vi "Sensorer_Cop.vi"() -> ()   [LabVIEW 2019]
uses:
  <vilib>/myRIO/Instrument Drivers/Onboard IO/AI/typedefs/AI Reference.ctl
  <vilib>/myRIO/Common/Instrument Driver Framework/Utilities/typedefs/myRIO Generic Hardware Reference.ctl
  <vilib>/myRIO/Common/Instrument Driver Framework/Utilities/typedefs/Hardware Version Enum.ctl
  <vilib>/myRIO/Common/Instrument Driver Framework/Utilities/typedefs/myRIO v1.0 Reference.ctl
  <vilib>/myRIO/Common/Instrument Driver Framework/Utilities/typedefs/Generic FPGA Reference.ctl
  <vilib>/myRIO/Common/Instrument Driver Framework/myRIO v1.0/AI/typedefs/AI Channels List.ctl
  <vilib>/myRIO/Common/Instrument Driver Framework/myRIO v1.0/AI/typedefs/AI Channels Enum.ctl
  <vilib>/myRIO/Common/Instrument Driver Framework/Utilities/typedefs/Analog Scaling Constants List.ctl
  <vilib>/myRIO/Common/Instrument Driver Framework/Utilities/typedefs/Analog Scaling Constants.ctl
  <vilib>/userDefined/High Color/nirio_resource_hc.ctl
  <vilib>/myRIO/Common/Instrument Driver Framework/Utilities/vis/Is FPGA Ref Available.vi
  <vilib>/myRIO/Common/Instrument Driver Framework/myRIO v1.0/AI/vis/myRIO v1.1 Open AI.vi
  <vilib>/myRIO/Instrument Drivers/Onboard IO/AI/vis/Read.vi
  <vilib>/myRIO/Common/Instrument Driver Framework/Utilities/vis/Validate Channels.vi
  <vilib>/myRIO/Common/Instrument Driver Framework/myRIO v1.0/AI/vis/myRIO v1.0 Reserve AI.vi
  <vilib>/myRIO/Common/Instrument Driver Framework/myRIO v1.0/AI/vis/myRIO v1.0 Build MUX Configuration AI.vi
  <vilib>/myRIO/Common/Instrument Driver Framework/myRIO v1.0/Resource Manager/vis/myRIO v1.0 Reserve Channel List.vi
  <vilib>/myRIO/Common/Instrument Driver Framework/myRIO v1.0/Resource Manager/vis/myRIO v1.0 Reserve Channel.vi
  <vilib>/myRIO/Common/Instrument Driver Framework/myRIO v1.0/Resource Manager/vis/myRIO v1.0 Unreserve Channel.vi
  <vilib>/myRIO/Common/Instrument Driver Framework/myRIO v1.0/Resource Manager/vis/myRIO v1.0 Build Mutex Name.vi
  <vilib>/Utility/VariantDataType/GetNumericInfo.vi
  <vilib>/Utility/error.llb/Error Cluster From Error Code.vi
  <vilib>/myRIO/Common/Instrument Driver Framework/myRIO v1.0/myRIO v1.1 Open.vi
  <vilib>/myRIO/Common/Instrument Driver Framework/myRIO v1.0/AI/vis/myRIO v1.0 Get Scaling Constants AI.vi
  <vilib>/myRIO/Common/Instrument Driver Framework/Utilities/vis/IO Manager.vi
  <vilib>/myRIO/Common/Instrument Driver Framework/Utilities/vis/Configuration Manager.vi
  <vilib>/myRIO/Common/Instrument Driver Framework/myRIO v1.0/myRIO v1.0 Close.vi
  <vilib>/myRIO/Common/Instrument Driver Framework/myRIO v1.0/AI/vis/myRIO v1.0 Read AI.vi
  <vilib>/myRIO/Express VI/Onboard IO/AI/AI Express VI.xnode
  <vilib>/myRIO/Instrument Drivers/Onboard IO/AI/vis/myRIO AI Open.xnode
  <vilib>/myRIO/Instrument Drivers/Onboard IO/AI/AI.lvlib
panel:
  in  "x Left":dbl[](array[numeric])
  in  "kal left":dbl
  in  "kal Right":dbl
  in  "x Right":dbl[](array[numeric])
  out "Cop Right":cluster{dbl[], dbl[]}(graph)
  out "Cop Left":cluster{dbl[], dbl[]}(graph)
  out "x(F.L)":dbl
  out "y(F.L)":dbl
  out "Sum (F.L)":dbl
  out "sum(F.R)":dbl
  out "y(F.R)":dbl
  out "x(F.R)":dbl
  in  "Cal(F.R)":dbl[](array[numeric])
  out "Kg (R)":dbl[](array[numeric])
  out "Sum(R)":dbl
  out "Sum(L)":dbl
  out "Kg(L)":dbl[](array[numeric])
  in  "Cal(F.L)":dbl[](array[numeric])
  out "Sensor 10":dbl=0.0038137989155123176 format="%0.5f"
  out "Axial(R)":T1(graph)
  out "Sensor 9":dbl=0.0038137989155123176 format="%0.5f"
  out "Axial(L)":T1(graph)
  out "Sensor 8":dbl=0.0038137989155123176 format="%0.5f"
  out "Back Right(F.R)":T1(graph)
  out "Sensor 7":dbl=0.0038137989155123176 format="%0.5f"
  out "Back Left(F.R)":T1(graph)
  out "Front Right(F.R)":T1(graph)
  out "Sensor 6":dbl=0.0038137989155123176 format="%0.5f"
  out "Front Left(F.R)":T1(graph)
  out "Sensor 5":dbl=0.0038137989155123176 format="%0.5f"
  out "Back Right(F.L)":T1(graph)
  out "Sensor 4":dbl=0.0038137989155123176 format="%0.5f"
  out "Back Left(F.L)":T1(graph)
  out "Sensor 3":dbl=0.0038137989155123176 format="%0.5f"
  out "Front  Right(F.L)":T1(graph)
  out "Sensor 2":dbl=0.0038137989155123176 format="%0.5f"
  in  "STOP SYSTEM":bool
  in  "ZERO ALL SENSORS":bool
  out "Sensor 1":dbl=0.0038137989155123176 format="%0.5f"
  out "Front  Left(F.L)":T1(graph)
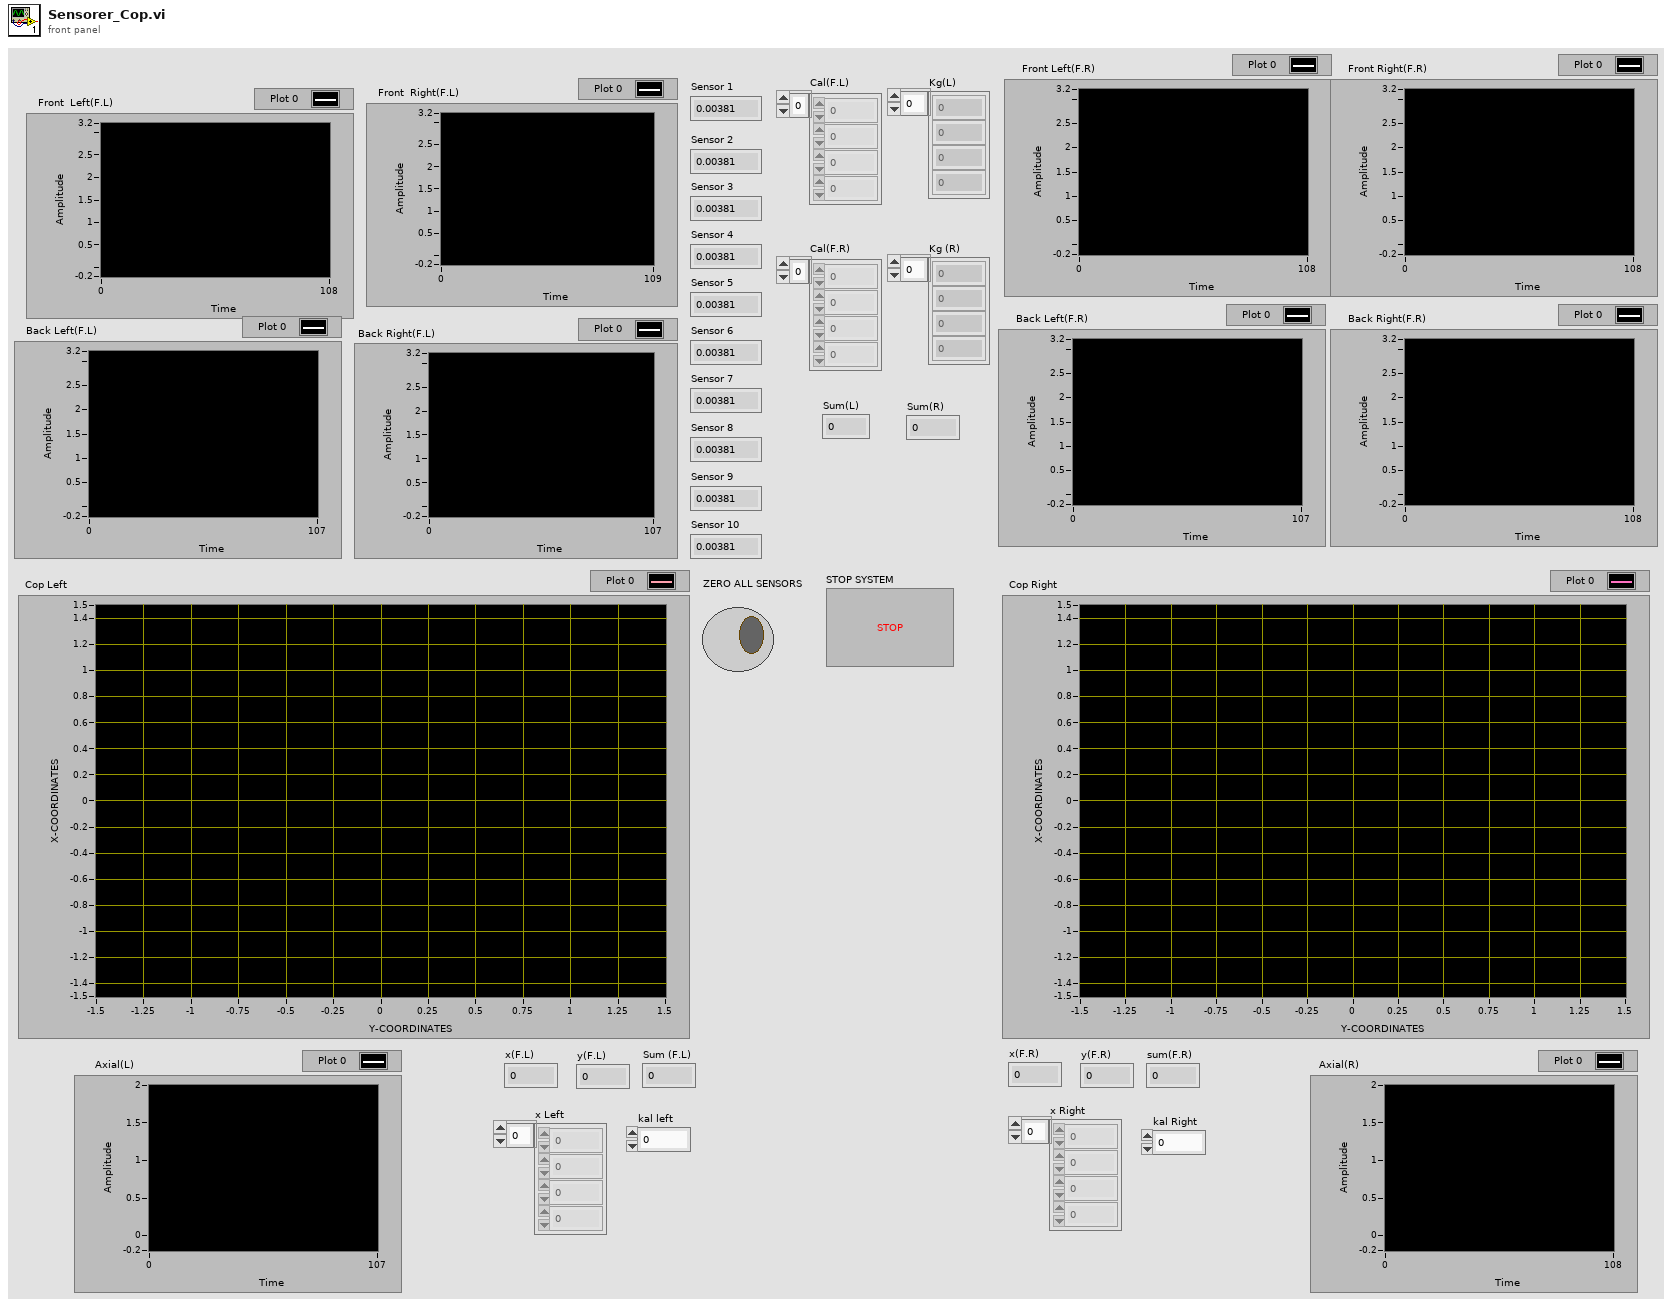
[diagram p1: front panel]
types:
  T1 = cluster{"Filtered x":dbl, "Sensor 1 (A/AI0 (Pin 3))":dbl}
  T2 = typedef "AI.lvlib/AI Reference.ctl" = cluster{"myRIO Reference":T3, "AI Channels List":T7, "AI Scaling Constants List":T9}
  T3 = typedef "myRIO Generic Hardware Reference.ctl" = cluster{"myRIO Model":T4, "myRIO Hardware Reference":T5}
  T4 = typedef "Hardware Version Enum.ctl" = enum16{"Unknown", "myRIO-1900", "myRIO-1950", "roboRIO", "NI ELVIS RIO CM", "ELVIS III"}
  T5 = typedef "myRIO v1.0 Reference.ctl" = cluster{"Generic FPGA Reference":T6, "Allow multiple opens":bool}
  T6 = typedef "Generic FPGA Reference.ctl" = refnum<k20>
  T7 = typedef "AI Channels List.ctl" = T8[]
  T8 = typedef "AI Channels Enum.ctl" = enum16{"Not Connected", "AudioIn/Left", "AudioIn/Right", "C/AI0", "C/AI1", "A/AI0", "A/AI1", "A/AI2", "A/AI3", "A/AI4", "A/AI5", "A/AI6", "A/AI7", "B/AI0", "B/AI1", "B/AI2", "B/AI3", "B/AI4", "B/AI5", "B/AI6", "B/AI7", "AI/AI0", "AI/AI1", "AI/AI2", "AI/AI3", "A/AI0 (DIFF)", "A/AI1 (DIFF)", "A/AI2 (DIFF)", "A/AI3 (DIFF)", "B/AI0 (DIFF)", "B/AI1 (DIFF)", "B/AI2 (DIFF)", "B/AI3 (DIFF)"}
  T9 = typedef "Analog Scaling Constants List.ctl" = T10[]
  T10 = typedef "Analog Scaling Constants.ctl" = cluster{"LSB Weight (Volts)":dbl, "Offset (Volts)":dbl, "Signed?":bool}
  T11 = typedef "nirio_resource_hc.ctl" = tag
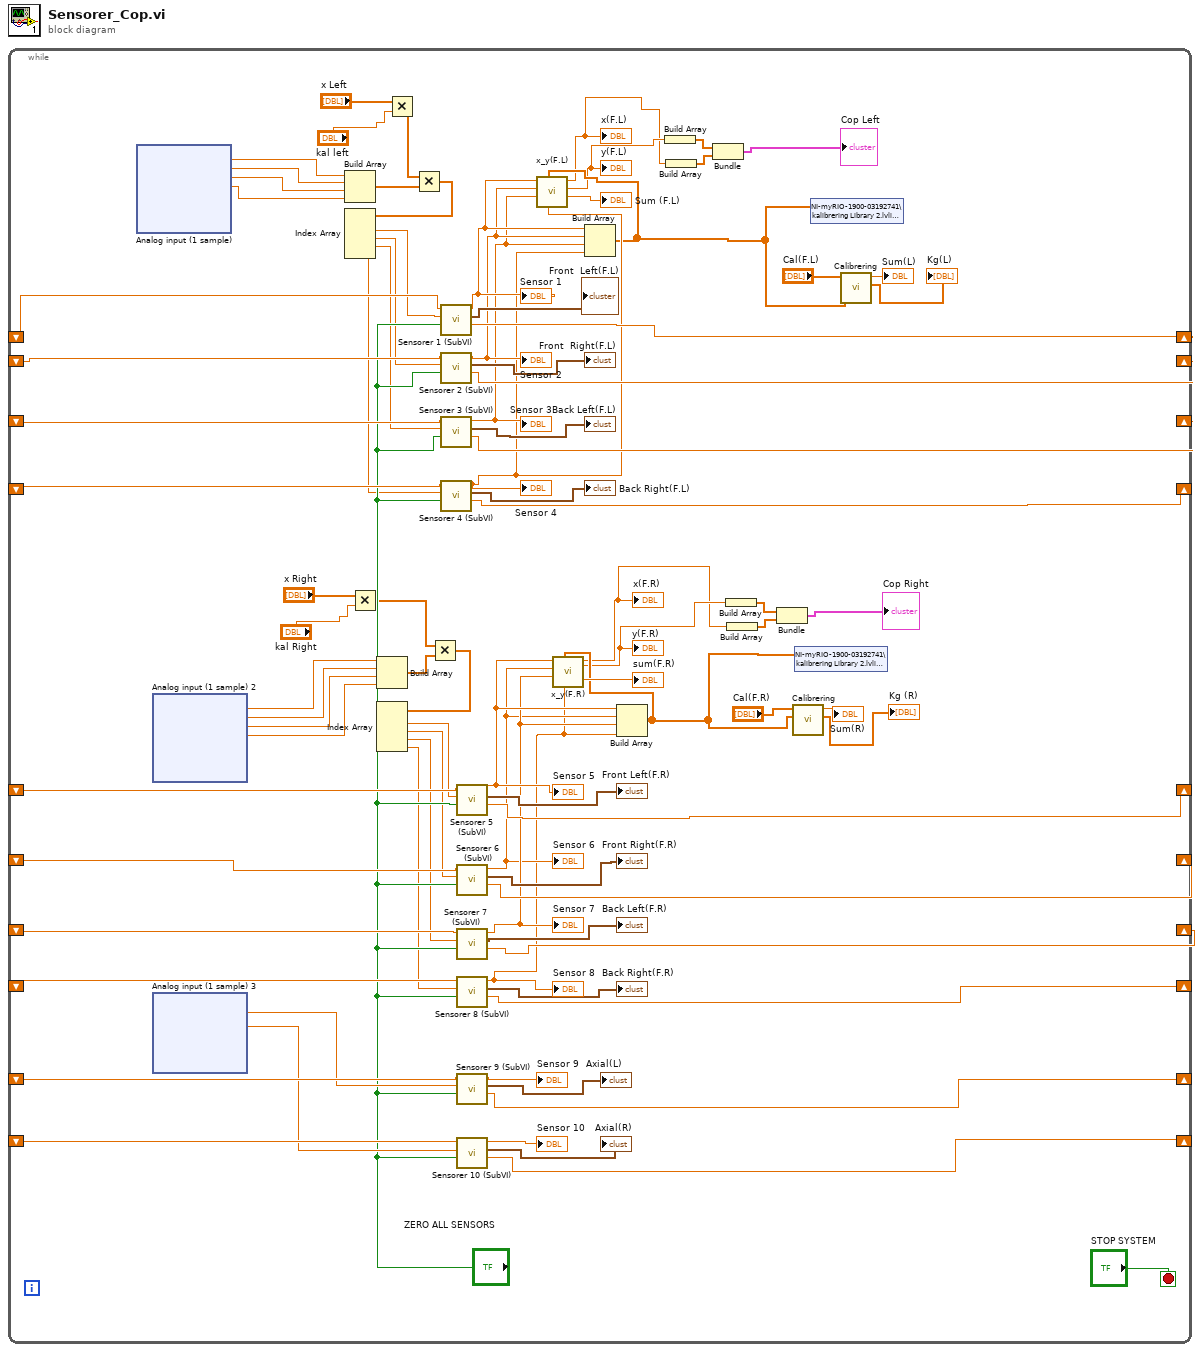
[diagram p0: block diagram]
diagram:
  n1 = while {
    shift-right: [w53] -> _
    shift-left: _ -> [w83]
    shift-right: [w51] -> _
    shift-left: _ -> [w82]
    shift-right: [w49] -> _
    shift-left: _ -> [w80]
    shift-right: [w52] -> _
    shift-left: _ -> [w78]
    shift-right: [w57] -> _
    shift-left: _ -> [w76]
    shift-right: [w56] -> _
    shift-left: _ -> [w74]
    shift-right: [w55] -> _
    shift-left: _ -> [w72]
    shift-right: [w54] -> _
    shift-left: _ -> [w70]
    shift-right: [w64] -> _
    shift-left: _ -> [w68]
    shift-right: [w58] -> _
    shift-left: _ -> [w63]
    stop <- "STOP SYSTEM" stop-if-true
    n2 = xnode "Analog input (1 sample)"() -> ("Sensor 1 (A/AI0 (Pin 3))"=w18:dbl, "Sensor 2 (A/AI1 (Pin 5))"=w17:dbl, "Sensor 3 (A/AI2 (Pin 7))"=w16:dbl, "Sensor 4 (A/AI3 (Pin 9))"=w15:dbl)  [unwired: 1 in, 1 out]
    n3 = xnode "Analog input (1 sample) 2"() -> ("Sensor 5 (B/AI0 (Pin 3))"=w28:dbl, "Sensor 6 (B/AI1 (Pin 5))"=w26:dbl, "Sensor 7 (B/AI2 (Pin 7))"=w4:dbl, "Sensor 8 (B/AI3 (Pin 9))"=w14:dbl)  [unwired: 1 in, 1 out]
    n4 = xnode "Analog input (1 sample) 3"() -> ("Sensor 9 (C/AI0 (AI0))"=w67:dbl, "Sensor 10 (C/AI1 (AI1))"=w62:dbl)  [unwired: 1 in, 1 out]
    n5 = Build Array(w18, w17, w16, w15) -> (w7:dbl[])
    n6 = Multiply(x="x Right", y="kal Right") -> (x*y=w22:dbl[])
    n7 = Build Array(w28, w26, w4, w14) -> (w31:dbl[])
    n8 = Multiply(x="x Left", y="kal left") -> (x*y=w6:dbl[])
    n9 = Multiply(x=w6, y=w7) -> (x*y=w5:dbl[])
    n10 = Index Array(array=w5) -> (element #1=w11:dbl, element #2=w10:dbl, element #3=w9:dbl, element #4=w8:dbl)  [unwired: 4 in]
    n11 = Multiply(x=w22, y=w31) -> (x*y=w29:dbl[])
    n12 = Index Array(array=w29) -> (element #1=w27:dbl, element #2=w25:dbl, element #3=w24:dbl, element #4=w23:dbl)  [unwired: 4 in]
    n13 = call "Sensorer 1 (SubVI).vi"("ZERO ALL SENSORS"="ZERO ALL SENSORS", "Sensor 3 (A/AI2(Pin7))"=w11, "Filtered x in"=w83) -> ("Filtered x out"=w53:dbl, "F.L Rear Leftt"=→"Front  Left(F.L)":T1, "Sensor 1"=w43:dbl)  [unwired: 6 in]
    "Sensor 1" <- w43
    n14 = call "Sensorer 2 (SubVI).vi"("ZERO ALL SENSORS"="ZERO ALL SENSORS", "Sensor 3 (A/AI2(Pin7))"=w10, "Filtered x in"=w82) -> ("Filtered x out"=w51:dbl, "F.L Rear Leftt"=→"Front  Right(F.L)":T1, "Sensor 1"=w42:dbl)  [unwired: 6 in]
    "Sensor 2" <- w42
    n15 = call "Sensorer 3 (SubVI).vi"("ZERO ALL SENSORS"="ZERO ALL SENSORS", "Sensor 3 (A/AI2(Pin7))"=w9, "Filtered x in"=w80) -> ("Filtered x out"=w49:dbl, "F.L Rear Leftt"=→"Back Left(F.L)":T1, "Sensor 1"=w41:dbl)  [unwired: 6 in]
    "Sensor 3" <- w41
    n16 = call "Sensorer 4 (SubVI).vi"("ZERO ALL SENSORS"="ZERO ALL SENSORS", "Sensor 3 (A/AI2(Pin7))"=w8, "Filtered x in"=w78) -> ("Filtered x out"=w52:dbl, "F.L Rear Leftt"=→"Back Right(F.L)":T1, "Sensor 1"=w40:dbl)  [unwired: 6 in]
    "Sensor 4" <- w40
    n17 = call "Sensorer 5 (SubVI).vi"("ZERO ALL SENSORS"="ZERO ALL SENSORS", "Sensor 3 (A/AI2(Pin7))"=w27, "Filtered x in"=w76) -> ("Filtered x out"=w57:dbl, "F.L Rear Leftt"=→"Front Left(F.R)":T1, "Sensor 1"=w47:dbl)  [unwired: 6 in]
    "Sensor 5" <- w47
    n18 = call "Sensorer 6 (SubVI).vi"("ZERO ALL SENSORS"="ZERO ALL SENSORS", "Sensor 3 (A/AI2(Pin7))"=w25, "Filtered x in"=w74) -> ("Filtered x out"=w56:dbl, "F.L Rear Leftt"=→"Front Right(F.R)":T1, "Sensor 1"=w45:dbl)  [unwired: 6 in]
    "Sensor 6" <- w45
    n19 = call "Sensorer 7 (SubVI).vi"("ZERO ALL SENSORS"="ZERO ALL SENSORS", "Sensor 3 (A/AI2(Pin7))"=w24, "Filtered x in"=w72) -> ("Filtered x out"=w55:dbl, "F.L Rear Leftt"=→"Back Left(F.R)":T1, "Sensor 1"=w46:dbl)  [unwired: 6 in]
    "Sensor 7" <- w46
    n20 = call "Sensorer 8 (SubVI).vi"("ZERO ALL SENSORS"="ZERO ALL SENSORS", "Sensor 3 (A/AI2(Pin7))"=w23, "Filtered x in"=w70) -> ("Filtered x out"=w54:dbl, "F.L Rear Leftt"=→"Back Right(F.R)":T1, "Sensor 1"=w44:dbl)  [unwired: 6 in]
    "Sensor 8" <- w44
    n21 = call "Sensorer 9 (SubVI).vi"("ZERO ALL SENSORS"="ZERO ALL SENSORS", "Sensor 3 (A/AI2(Pin7))"=w67, "Filtered x in"=w68) -> ("Filtered x out"=w64:dbl, "F.L Rear Leftt"=→"Axial(L)":T1, "Sensor 1"=→"Sensor 9":dbl)  [unwired: 6 in]
    n22 = call "Sensorer 10 (SubVI).vi"("ZERO ALL SENSORS"="ZERO ALL SENSORS", "Sensor 3 (A/AI2(Pin7))"=w62, "Filtered x in"=w63) -> ("Filtered x out"=w58:dbl, "F.L Rear Leftt"=→"Axial(R)":T1, "Sensor 1"=→"Sensor 10":dbl)  [unwired: 6 in]
    n23 = Build Array(w43, w42, w41, w40) -> (w32:dbl[])
    n24 = call "x_y(F.L).vi"("Sensor 4"=w40, "Array"=w32, "Sensor 3"=w41, "Sensor 2"=w42, "Sensor 1"=w43) -> ("Sum (F.L)"=→"Sum (F.L)":dbl, "y(F.L)"=w3:dbl, "x(F.L)"=w2:dbl)  [unwired: 4 in]
    "y(F.L)" <- w3
    "x(F.L)" <- w2
    n25 = Build Array(w47, w45, w46, w44) -> (w38:dbl[])
    n26 = call "x_y(F.R).vi"("Sensor 8"=w44, "Array"=w38, "Sensor 7"=w46, "Sensor 6"=w45, "Sensor 5"=w47) -> ("Sum(F.R)"=→"sum(F.R)":dbl, "y(F.R)"=w20:dbl, "x(F.R)"=w19:dbl)  [unwired: 4 in]
    "x(F.R)" <- w19
    "y(F.R)" <- w20
    n27 = Build Array(w3) -> (w37:dbl[])
    n28 = Build Array(w2) -> (w34:dbl[])
    n29 = Bundle(w37, w34) -> (→"Cop Left":cluster{dbl[], dbl[]})  [unwired: 1 in]
    n30 = Build Array(w20) -> (w36:dbl[])
    n31 = Build Array(w19) -> (w35:dbl[])
    n32 = Bundle(w36, w35) -> (→"Cop Right":cluster{dbl[], dbl[]})  [unwired: 1 in]
    n33 = call "Calibrering.vi"("Array"=w38, "Cal(F.L)"="Cal(F.R)") -> ("Kg"=→"Kg (R)":dbl[], "sum"=→"Sum(R)":dbl)  [unwired: 8 in]
    n34 = shared-variable "NI-myRIO-1900-03192741\\kalibrering Library 2.lvlib\\Variable2"(w38) -> ()  [unwired: 1 in, 1 out]
    n35 = shared-variable "NI-myRIO-1900-03192741\\kalibrering Library 2.lvlib\\Variable2"(w32) -> ()  [unwired: 1 in, 1 out]
    n36 = call "Calibrering.vi"("Array"=w32, "Cal(F.L)"="Cal(F.L)") -> ("Kg"=→"Kg(L)":dbl[], "sum"=→"Sum(L)":dbl)  [unwired: 8 in]
  }
